vi "Swipe.vi"() -> ()   [LabVIEW 2010]
uses:
  <vilib>/Utility/miscctls.llb/LVPointTypeDef.ctl
  <vilib>/Utility/inputDevices.llb/mouseAcquire.vi
  <vilib>/addons/control/pid/pid.llb/PID (DBL).vi
  <vilib>/Analysis/NI_AALBase.lvlib
  <vilib>/addons/control/pid/NI_PID_pid.lvlib
panel:
  out "mean":i32=88
  in  "Page Swipe Sensitivity":i32=400
  in  "Bottom Page":i16
  in  "Top Page":i16=3
  in  "Current Page":i16
  out "Bounds.Right":i16=1280
  out "Coords":T1={"Horizontal"=378, "Vertical"=449, "Scrolling"=0}
  out "Boolean 2":bool
  out "Swipe Start":T1={"Horizontal"=604, "Vertical"=459, "Scrolling"=0}
  in  "Sensitivity":i32=100
  out "axis info":T1={"Horizontal"=107, "Vertical"=143, "Scrolling"=0}
  out "Boolean":bool
  in  "stop":bool
  # "Page 1"
  # "Page0"
  # "Page 2"
  # "Page 3"
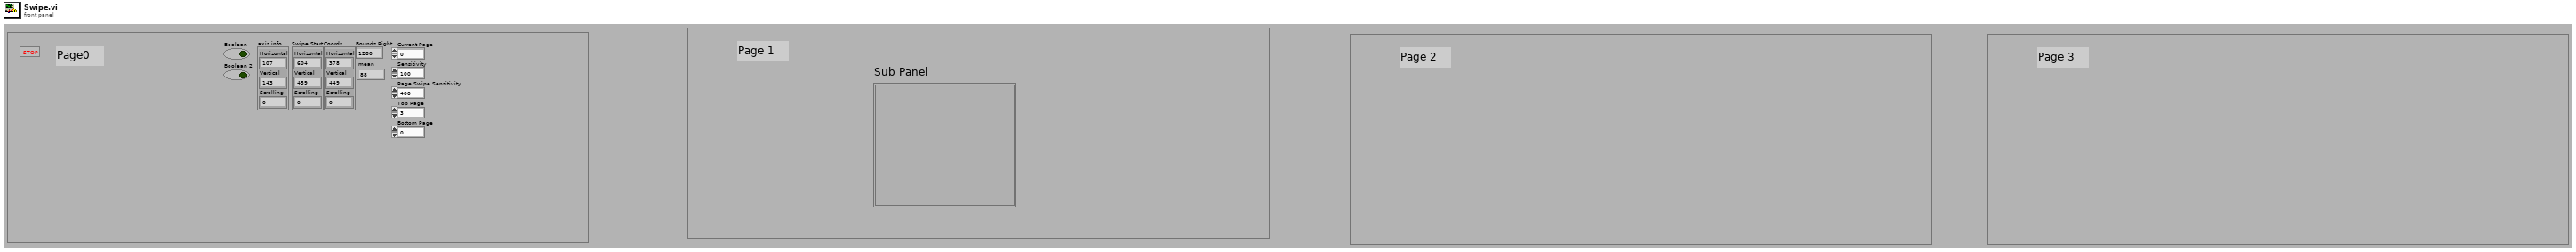
[diagram p1: front panel]
types:
  T1 = cluster{"Horizontal":i32, "Vertical":i32, "Scrolling":i32}
  T2 = typedef "LVPointTypeDef.ctl" = cluster{"Horizontal":i16, "Vertical":i16}
  T3 = cluster{"proportional gain (Kc)":dbl, "integral time (Ti, min)":dbl, "derivative time (Td, min)":dbl}
  T4 = typedef "LVRectTypeDef.ctl" = cluster{"left":i16, "top":i16, "right":i16, "bottom":i16}
  T5 = typedef "LVAllMonitorsDisplayTypeDef.ctl" = cluster{"Bounds":cluster{"Left":i16, "Top":i16, "Right":i16, "Bottom":i16}, "Depth":i16}[]
  T6 = cluster{"Bounds":cluster{"Left":i16, "Top":i16, "Right":i16, "Bottom":i16}, "Depth":i16}
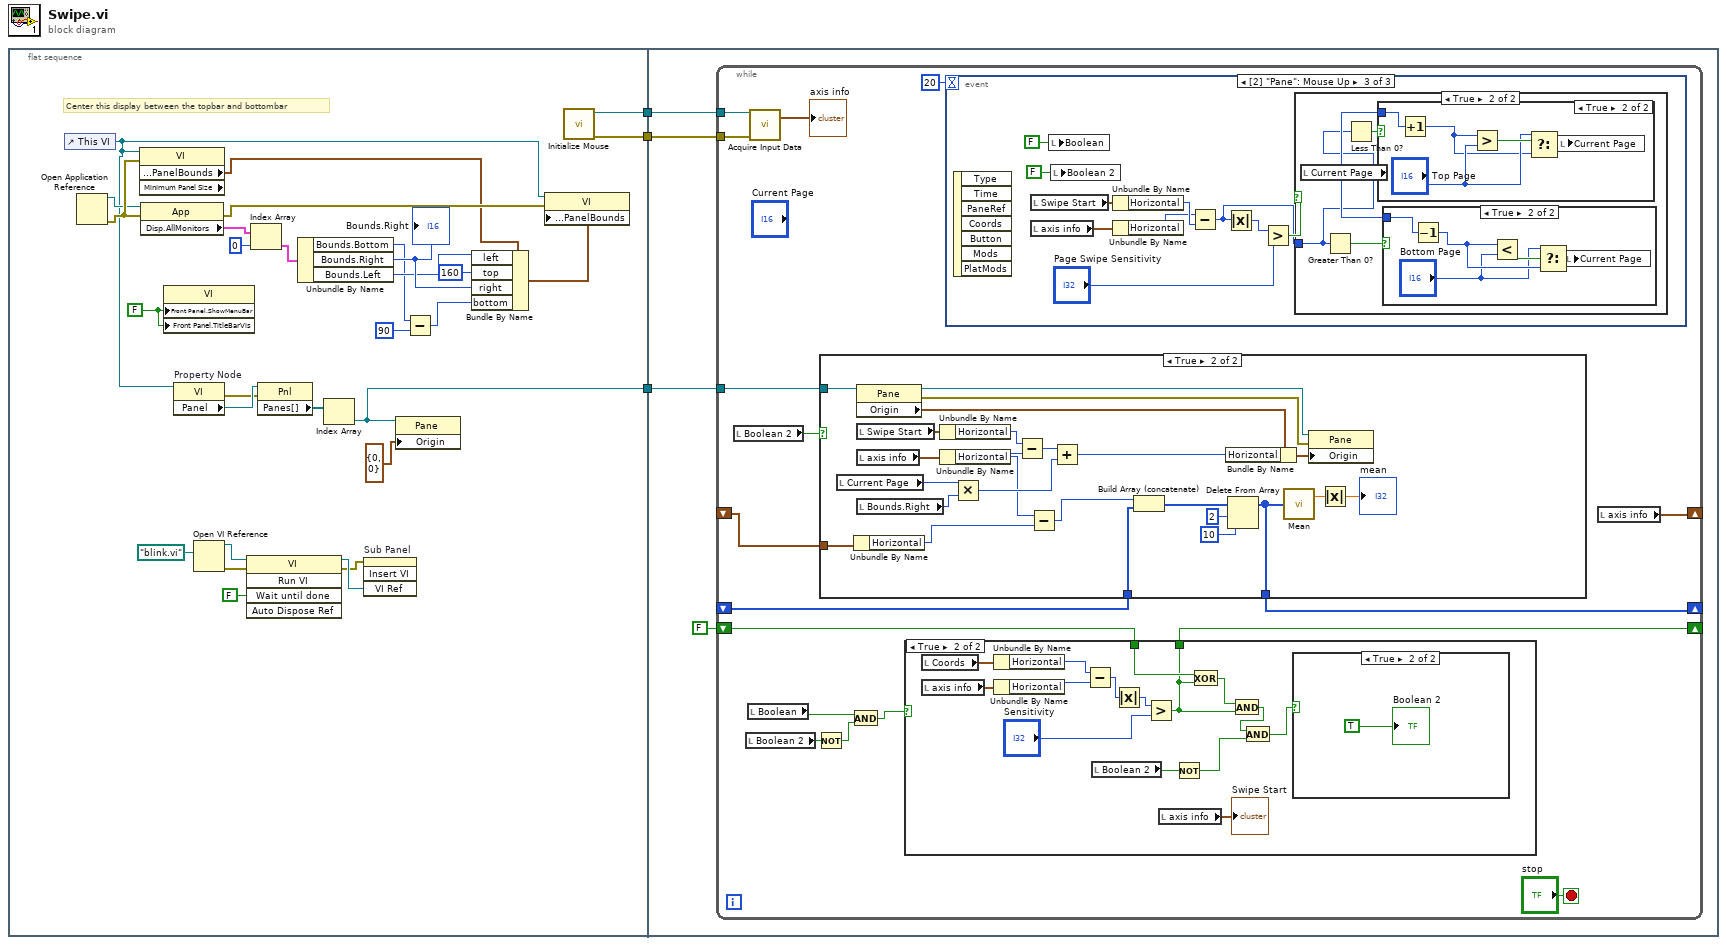
[diagram p0: block diagram]
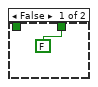
[diagram p2: hidden frame]
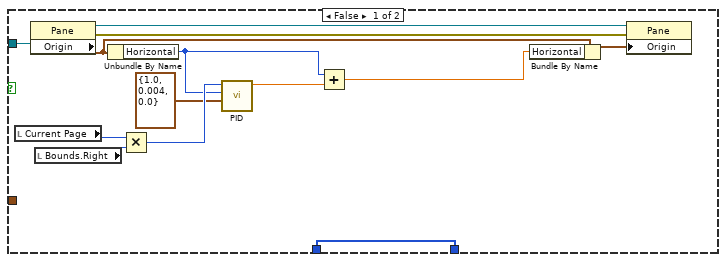
[diagram p4: hidden frame]
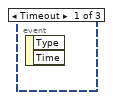
[diagram p5: hidden frame]
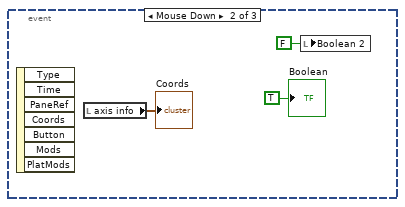
[diagram p6: hidden frame]
diagram:
  n1 = flat-sequence {
    tunnel: [w13] -> w3
    tunnel: [w11] -> w2
    tunnel: [w10] -> w1
    tunnel: w3 -> [w36]
    tunnel: w2 -> [w35]
    tunnel: w1 -> [w34]
    frame #0 {
      w12 = FALSE ("Front Panel Window:Show Menu Bar")
      # "Center this display between the topbar and bottombar"
      n2 = control-ref of="This VI"() -> (w14:refnum<vi>)
      n3 = Open Application Reference() -> (0:w24:errorcluster, 3:w15:refnum<vi>)  [unwired: 4 in]
      n4 = property class="VI" props=["Front Panel.PanelBounds", "Minimum Panel Size"](reference=w14, error in=w24) -> ("Front Panel.PanelBounds"=w27:T4)  [unwired: 3 out]
      n5 = property class="App"(reference=w15, error in=w24) -> (error out=w29:errorcluster, "Disp.AllMonitors"=w31:T5)  [unwired: 1 out]
      n6 = property class="VI"("Front Panel.ShowMenuBar"=w12, "Front Panel.TitleBarVis"=w12) -> ()  [unwired: 2 in, 2 out]
      n7 = property on="Property Node" class="VI"(reference=w14) -> (error out=w18:errorcluster, "Panel"=w19:refnum<vi>)  [unwired: 1 in, 1 out]
      n8 = Open VI Reference(vi path=path "blink.vi") -> (vi reference=w7:refnum<vi>, error out=w4:errorcluster)  [unwired: 5 in]
      n9 = invoke class="VI" method="Run VI"(reference=w7, error in=w4, "Wait until done"=FALSE ("Wait Until Done")) -> (reference out=w6:refnum<vi>, error out=w5:errorcluster)  [unwired: 2 in, 3 out]
      n10 = Index Array(array=w31, index=0) -> (element=w32:T6)
      n11 = property class="Pnl"(reference=w19, error in=w18) -> ("Panes[]"=w17:refnum<vi>[])  [unwired: 2 out]
      n12 = Unbundle By Name(w32) -> ("Bounds.Bottom"=w22:i16, "Bounds.Right"=w26:i16, "Bounds.Left"=w25:i16)
      "Bounds.Right" <- w26
      n13 = Index Array "Index Array"(array=w17) -> (element=w13:refnum<vi>)  [unwired: 1 in]
      n14 = invoke on="Sub Panel" class="SubPanel" method="Insert VI"(error in=w5, "VI Ref"=w6) -> ()  [unwired: 2 in, 4 out]
      n15 = property class="Pane"(reference=w13, "Origin"=T2 {"Horizontal"=0, "Vertical"=0}) -> ()  [unwired: 1 in, 2 out]
      n16 = Subtract(x=w22, y=i16 90) -> (x-y=w20:i16)
      n17 = Bundle By Name(cluster=w27, "left"=w25, "top"=i16 160, "right"=w26, "bottom"=w20) -> (w28:T4)
      n18 = property class="VI"(reference=w14, error in=w29, "Front Panel.PanelBounds"=w28) -> ()  [unwired: 2 out]
      n19 = call <vilib>:"Initialize Mouse.vi"() -> ("error out"=w10:errorcluster, "device ID"=w11:refnum<k1>)  [unwired: 1 in, 9 out]
    }
    frame #1 {
      n20 = while {
        tunnel: w36 -> [w52]
        tunnel: w35 -> [w50]
        tunnel: w34 -> [w49]
        shift-right: [w45] -> _
        shift-left: FALSE -> [w46]
        shift-right: [w40] -> _
        shift-left: _ -> [w39]
        shift-right: [w38] -> _
        shift-left: _ -> [w37]
        stop <- "stop" stop-if-true
        n21 = local read "Boolean 2"() -> (w47:bool)
        n22 = local read "Boolean 2"() -> (w43:bool)
        n23 = local read "Boolean"() -> (w44:bool)
        n24 = call-poly <vilib>:"Acquire Input Data.vi"("device ID"=w50, "error in (no error)"=w49) -> ("axis info"=→"axis info":T1)  [unwired: 14 in, 3 out]
        n25 = Not(x=w43) -> (.not. x?=w42:bool)
        n26 = case shown="True" w47 {
          tunnel: w52 -> [w83 w102]
          tunnel: [w76 w90] -> w40
          tunnel: w39 -> [w76 w91]
          tunnel: w37 -> [_ w87]
          frame False {
            n27 = local read "Current Page"() -> (w78:i16)
            n28 = property class="Pane"(reference=w83) -> (reference out=w82:refnum<vi>, error out=w81:errorcluster, "Origin"=w79:T2)  [unwired: 1 in]
            n29 = local read "Bounds.Right"() -> (w77:i16)
            n30 = Unbundle By Name(w79) -> ("Horizontal"=w73:i16)
            n31 = Multiply(x=w78, y=w77) -> (x*y=w75:i16)
            n32 = call-poly <vilib>:"PID.vi"("PID gains"=T3 {"proportional gain (Kc)"=1.0, "integral time (Ti, min)"=0.004, "derivative time (Td, min)"=0.0}, "process variable"=w73, "setpoint"=w75) -> ("output"=w72:dbl)  [unwired: 7 in, 1 out]
            n33 = Add(x=w73, y=w72) -> (x+y=w71:dbl)
            n34 = Bundle By Name(cluster=w79, "Horizontal"=w71) -> (w80:T2)
            n35 = property class="Pane"(reference=w82, error in=w81, "Origin"=w80) -> ()  [unwired: 2 out]
          }
          frame True {
            n36 = local read "Current Page"() -> (w98:i16)
            n37 = Unbundle By Name(w87) -> ("Horizontal"=w85:i32)
            n38 = property class="Pane"(reference=w102) -> (reference out=w104:refnum<vi>, error out=w103:errorcluster, "Origin"=w101:T2)  [unwired: 1 in]
            n39 = local read "Swipe Start"() -> (w105:T1)
            n40 = local read "axis info"() -> (w96:T1)
            n41 = local read "Bounds.Right"() -> (w99:i16)
            n42 = Unbundle By Name(w105) -> ("Horizontal"=w106:i32)
            n43 = Unbundle By Name(w96) -> ("Horizontal"=w86:i32)
            n44 = Multiply(x=w98, y=w99) -> (x*y=w97:i16)
            n45 = Subtract(x=w106, y=w86) -> (x-y=w92:i32)
            n46 = Subtract(x=w86, y=w85) -> (x-y=w84:i32)
            n47 = Add(x=w92, y=w97) -> (x+y=w100:i32)
            n48 = Build Array (concatenate)(w84, w91) -> (w93:i32[])
            n49 = Bundle By Name(cluster=w101, "Horizontal"=w100) -> (w107:T2)
            n50 = Delete From Array(array=w93, length=2, index=10) -> (array with subset deleted=w90:i32[])  [unwired: 1 out]
            n51 = call <vilib>:"Mean.vi"("X"=w90) -> ("mean"=w89:dbl)  [unwired: 1 out]
            n52 = property class="Pane"(reference=w104, error in=w103, "Origin"=w107) -> ()  [unwired: 2 out]
            n53 = Absolute Value(x=w89) -> (abs(x)=→"mean":dbl)
          }
        }
        n54 = And(x=w44, y=w42) -> (x .and. y?=w41:bool)
        n55 = case shown="True" w41 {
          tunnel: [FALSE w56] -> w45
          tunnel: w46 -> [_ w63]
          frame False {
          }
          frame True {
            n56 = local read "Coords"() -> (w68:T1)
            n57 = local read "axis info"() -> (w66:T1)
            n58 = Unbundle By Name(w68) -> ("Horizontal"=w69:i32)
            n59 = Unbundle By Name(w66) -> ("Horizontal"=w67:i32)
            n60 = Subtract(x=w69, y=w67) -> (x-y=w62:i32)
            n61 = local read "Boolean 2"() -> (w58:bool)
            n62 = Absolute Value(x=w62) -> (abs(x)=w61:i32)
            n63 = Greater?(x=w61, y="Sensitivity") -> (0:w56:bool)
            n64 = local read "axis info"() -> (→"Swipe Start":T1)
            n65 = Not(x=w58) -> (.not. x?=w59:bool)
            n66 = Exclusive Or(1:w56, 2:w63) -> (0:w64:bool)
            n67 = And(x=w64, y=w56) -> (x .and. y?=w60:bool)
            n68 = And(x=w60, y=w59) -> (x .and. y?=w57:bool)
            n69 = case shown="True" w57 {
              frame False {
              }
              frame True {
                "Boolean 2" <- TRUE
              }
            }
          }
        }
        n70 = event shown="[2] \"Pane\": Mouse Up" {
          selector: _ -> [_ _ _]
          dyn-events: _ -> [_ _ _]
          timeout: 20 -> [_ _ _]
          event Timeout {
            n71 = event-data() -> ()  [unwired: 1 in, 2 out]
          }
          event Mouse Down {
            n72 = event-data() -> ()  [unwired: 1 in, 7 out]
            n73 = local read "axis info"() -> (→"Coords":T1)
            n74 = local write "Boolean 2"(FALSE ("Boolean 2")) -> ()
            "Boolean" <- TRUE
          }
          event Mouse Up {
            n75 = event-data() -> ()  [unwired: 1 in, 7 out]
            n76 = local read "Swipe Start"() -> (w118:T1)
            n77 = local read "axis info"() -> (w115:T1)
            n78 = local write "Boolean"(FALSE ("Boolean")) -> ()
            n79 = local write "Boolean 2"(FALSE ("Boolean 2")) -> ()
            n80 = Unbundle By Name(w118) -> ("Horizontal"=w117:i32)
            n81 = Unbundle By Name(w115) -> ("Horizontal"=w116:i32)
            n82 = Subtract(x=w116, y=w117) -> (x-y=w113:i32)
            n83 = Absolute Value(x=w113) -> (abs(x)=w111:i32)
            n84 = Greater?(x=w111, y="Page Swipe Sensitivity") -> (0:w114:bool)
            n85 = case shown="True" w114 {
              tunnel: w113 -> [_ w121]
              frame False {
              }
              frame True {
                n86 = local read "Current Page"() -> (w124:i16)
                n87 = Greater Than 0?(x=w121) -> (x > 0?=w123:bool)
                n88 = Less Than 0?(x=w121) -> (x < 0?=w122:bool)
                n89 = case shown="True" w122 {
                  tunnel: w124 -> [_ w129]
                  frame False {
                  }
                  frame True {
                    n90 = Increment(x=w129) -> (x+1=w126:i16)
                    n91 = Greater?(x=w126, y="Top Page") -> (0:w128:bool)
                    n92 = Select(t="Top Page", s=w128, f=w126) -> (s? t:f=w125:i16)
                    n93 = local write "Current Page"(w125) -> ()
                  }
                }
                n94 = case shown="True" w123 {
                  tunnel: w124 -> [_ w134]
                  frame False {
                  }
                  frame True {
                    n95 = Decrement(x=w134) -> (x-1=w132:i16)
                    n96 = Less?(x=w132, y="Bottom Page") -> (x < y?=w133:bool)
                    n97 = Select(t="Bottom Page", s=w133, f=w132) -> (s? t:f=w130:i16)
                    n98 = local write "Current Page"(w130) -> ()
                  }
                }
              }
            }
          }
        }
        n99 = local read "axis info"() -> (w38:T1)
      }
    }
  }
